vi "Reject rel times before reset.vi"(10 "Timestamps (ms)":dbl[](array[numeric])) -> (3 "Keep":bool[](array[boolean]))   [LabVIEW 2013]
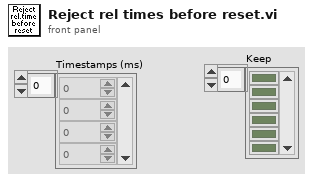
[diagram p1: front panel]
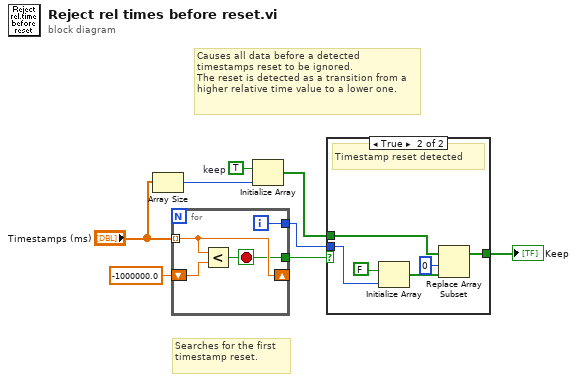
[diagram p0: block diagram]
diagram:
  w6 = TRUE  # keep
  # "Searches for the first timestamp reset."
  # "Causes all data before a detected timestamps reset to be ignored.\nThe reset is detected as a transition from a higher relative time value to a lower one."
  n1 = Array Size(array="Timestamps (ms)") -> (size(s)=w5:i32)
  n2 = for {
    tunnel: "Timestamps (ms)" -> [w12] mode=indexing
    shift-right: [w12] -> _
    shift-left: -1000000.0 ("String") -> [w11]
    tunnel: [w10] -> w4
    tunnel: [w9] -> w3
    i -> [w10]
    stop <- w9 stop-if-true
    n3 = Less?(x=w12, y=w11) -> (x < y?=w9:bool)
  }
  n4 = Initialize Array(w6, w5) -> (w7:bool[])
  n5 = case shown="True" w3 {
    tunnel: w4 -> [_ w18]
    tunnel: w7 -> [w13 w17]
    tunnel: [w13 w14] -> w8
    frame False {
      # "Keep all"
    }
    frame True {
      # "Timestamp reset detected"
      n6 = Initialize Array(FALSE ("No test header file"), w18) -> (w16:bool[])
      n7 = Replace Array Subset(array=w17, new element=w16, index=0) -> (w14:bool[])
    }
  }
  "Keep" <- w8
